vi "cTOf.vi"(11 "Fahrenheit":dbl) -> (3 "Numeric":dbl)   [LabVIEW 2017]
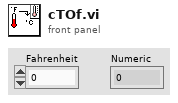
[diagram p1: front panel]
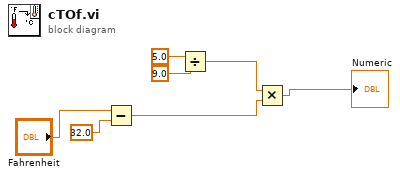
[diagram p0: block diagram]
diagram:
  n1 = Subtract(x="Fahrenheit", y=32.0 ("x")) -> (x-y=w3:dbl)
  n2 = Divide(x=5.0, y=9.0) -> (x/y=w4:dbl)
  n3 = Multiply(x=w4, y=w3) -> (x*y=→"Numeric":dbl)
